vi "Get Date String For Current File.vi"(11 "Time to Rotate":timestamp format="%<%H:%M>T") -> ()   [LabVIEW 2020, in "LV Log.lvlib" / "Rotating Daily File Sink.lvclass"]
uses:
  Rotating Daily File Sink.lvclass
panel:
  out "date string":string
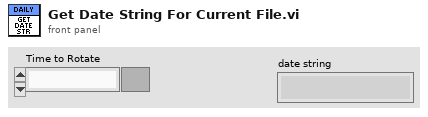
[diagram p1: front panel]
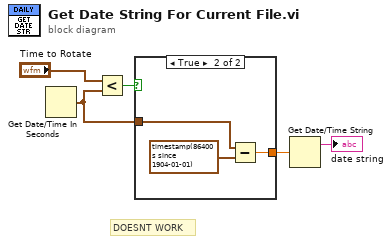
[diagram p0: block diagram]
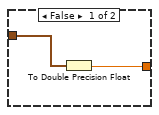
[diagram p2: hidden frame]
diagram:
  # "DOESNT WORK"
  n1 = Get Date/Time In Seconds() -> (seconds since 1Jan1904=w2:timestamp)
  n2 = Less?(x="Time to Rotate", y=w2) -> (x < y?=w3:bool)
  n3 = case shown="True" w3 {
    tunnel: w2 -> [w7 w9]
    tunnel: [w6 w8] -> w4
    frame False {
      n4 = To Double Precision Float(number=w7) -> (double precision float=w6:dbl)
    }
    frame True {
      n5 = Subtract(x=w9, y=timestamp(86400 s since 1904-01-01)) -> (x-y=w8:dbl)
    }
  }
  n6 = Get Date/Time String(seconds (now)=w4) -> (date string=→"date string":string)  [unwired: 2 in, 1 out]
